vi "範圍內全部點.vi"() -> ()   [LabVIEW 2015]
panel:
  out "first y":dbl=-1000.0
  out "first x":dbl=-1000.0
  out "XY Graph":cluster{dbl[], dbl[]}(graph)
  out "執行次數":i32
  out "Boolean":bool
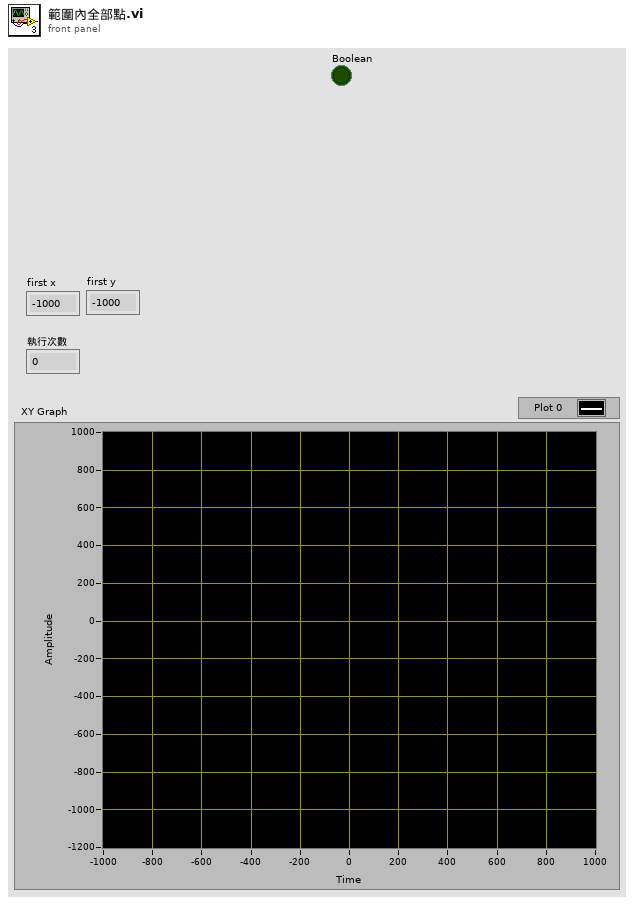
[diagram p1: front panel]
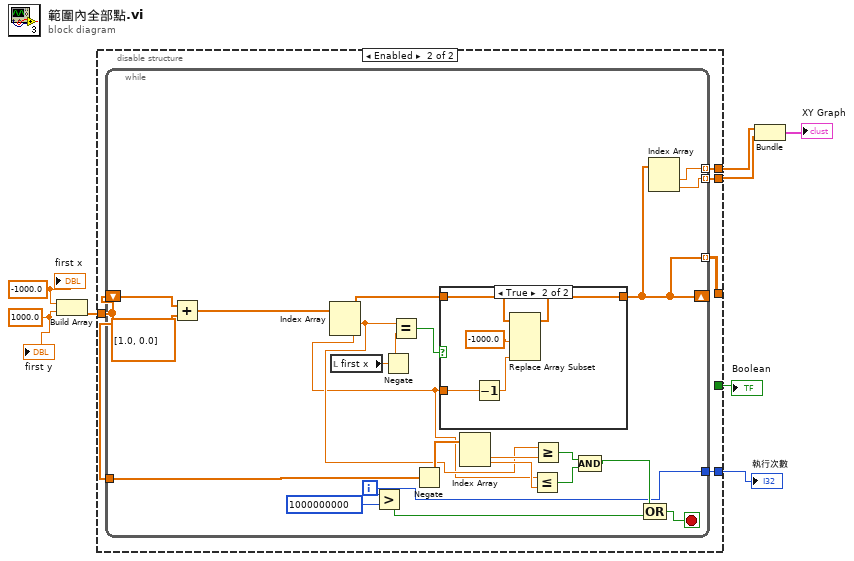
[diagram p0: block diagram]
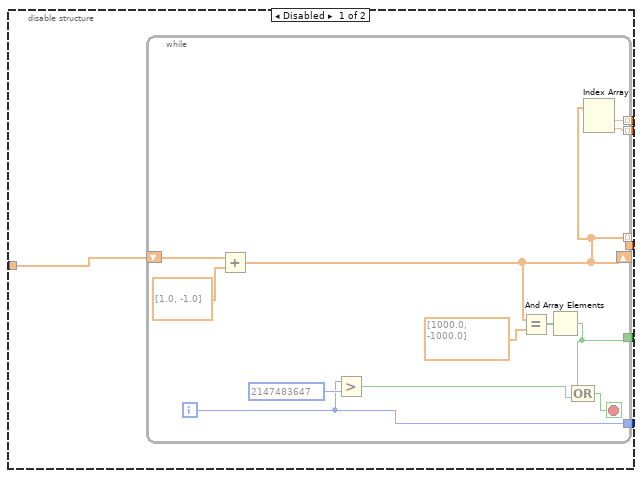
[diagram p2: hidden frame]
diagram:
  w1 = 1000.0
  w3 = -1000.0
  n1 = Build Array(w3, w1) -> (w2:dbl[])
  n2 = disable-structure shown="Enabled" {
    disable-tunnel: [w13 _] -> w8
    disable-tunnel: [w12 w27] -> w7
    disable-tunnel: [w11 w30] -> w6
    disable-tunnel: [w10 w29] -> w5
    disable-tunnel: w2 -> [w9 w28]
    disable-tunnel: [_ w26] -> _
    frame Disabled {
      n3 = while {
        shift-right: [w16] -> _
        shift-left: w9 -> [w24]
        tunnel: [w16] -> _ mode=indexing
        tunnel: [w18] -> w13
        tunnel: [w17] -> w12
        tunnel: [w15] -> w11 mode=indexing
        tunnel: [w14] -> w10 mode=indexing
        i -> [w17]
        stop <- w21 stop-if-true
        n4 = Add(x=w24, y=dbl[] [1.0, -1.0]) -> (x+y=w16:dbl[])
        n5 = Greater?(x=w17, y=2147483647) -> (0:w22:bool)
        n6 = Equal?(x=w16, y=dbl[] [1000.0, -1000.0]) -> (x = y?=w19:bool[])
        n7 = And Array Elements(Boolean array=w19) -> (logical AND=w18:bool)
        n8 = Compound Arithmetic op=OR(w18, w22) -> (w21:bool)
        n9 = Index Array(array=w16) -> (element #1=w15:dbl, element #2=w14:dbl)  [unwired: 2 in]
      }
    }
    frame Enabled {
      n10 = while {
        shift-right: [w31] -> _
        shift-left: w28 -> [w51]
        tunnel: [w45] -> w30 mode=indexing
        tunnel: [w44] -> w29 mode=indexing
        tunnel: w28 -> [w40]
        tunnel: [w32] -> w27
        tunnel: [w31] -> w26 mode=indexing
        i -> [w32]
        stop <- w43 stop-if-true
        n11 = Add(x=w51, y=dbl[] [1.0, 0.0]) -> (x+y=w46:dbl[])
        n12 = Index Array(array=w46) -> (element #1=w35:dbl, element #2=w34:dbl)  [unwired: 2 in]
        n13 = local read "first x"() -> (w49:dbl)
        n14 = Greater?(x=w32, y=1000000000) -> (0:w42:bool)
        n15 = Negate(x=w49) -> (-x=w48:dbl)
        n16 = Equal?(x=w35, y=w48) -> (x = y?=w47:bool)
        n17 = Negate(x=w40) -> (-x=w41:dbl[])
        n18 = case shown="True" w47 {
          tunnel: w46 -> [w53 w58]
          tunnel: [w53 w56] -> w31
          tunnel: w34 -> [_ w54]
          frame False {
          }
          frame True {
            n19 = Decrement(x=w54) -> (x-1=w55:dbl)
            n20 = Replace Array Subset(array=w58, new element #1=-1000.0 ("new element/subarray"), new element #2=w55) -> (w56:dbl[])  [unwired: 2 in]
          }
        }
        n21 = Index Array(array=w41) -> (element #1=w36:dbl, element #2=w37:dbl)  [unwired: 2 in]
        n22 = Less Or Equal?(x=w34, y=w37) -> (x <= y?=w38:bool)
        n23 = Greater Or Equal?(x=w35, y=w36) -> (x >= y?=w39:bool)
        n24 = Compound Arithmetic op=AND(w39, w38) -> (w33:bool)
        n25 = Compound Arithmetic op=OR(w33, w42) -> (w43:bool)
        n26 = Index Array(array=w31) -> (element #1=w45:dbl, element #2=w44:dbl)  [unwired: 2 in]
      }
    }
  }
  "Boolean" <- w8
  "執行次數" <- w7
  n27 = Bundle(w6, w5) -> (→"XY Graph":cluster{dbl[], dbl[]})  [unwired: 1 in]
  "first x" <- w3
  "first y" <- w1
